vi "publishCurrentState.vi"(8 "error in (no error)":errorcluster, 11 "ElectrometerController in":refnum<class "ElectrometerController.lvclass">) -> (0 "error out":errorcluster, 3 "ElectrometerController out":refnum<class "ElectrometerController.lvclass">)   [LabVIEW 2016, in "ElectrometerController.lvclass"]
uses:
  ElectrometerController.lvclass
  ts_sallv_calibrationelectrometer/DataTypes/logevent_DetailedState.ctl
  ElectrometerController.lvclass/ElectrometerController.ctl
  ts_electrometeruserevents/PubSubDataEvent/PubSubDataEvent.lvclass/PubSubDataEvent.ctl
  Electrometer/State/ElectrometerState.lvclass
  ts_electrometeruserevents/PubSubDataEvent/PubSubDataEvent.lvclass
  ts_sallv_calibrationelectrometer/SALLV_calibrationElectrometer.lvlib
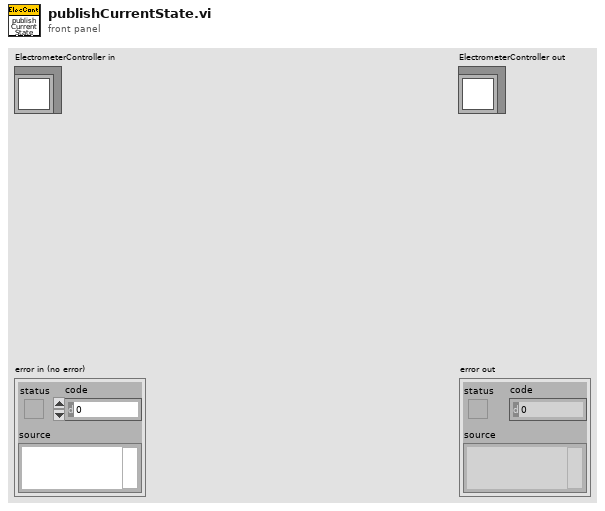
[diagram p1: front panel]
types:
  T1 = typedef "SALLV_calibrationElectrometer.lvlib/logevent_DetailedState.ctl" = cluster{"detailedState":u16, "electId":i16, "priority":i32}
  T2 = typedef "ElectrometerTypedefs.lvlib/PubDataEvents.ctl" = cluster{"ErrorCode":refnum<user-event>, "Heartbeat":refnum<user-event>, "LoopTime_ms":refnum<user-event>, "LoopTimeOutOfRange":refnum<user-event>, "RejectedCommand":refnum<user-event>, "SummaryState":refnum<user-event>, "Timestamp":refnum<user-event>, "AppliedSettingsMatchStart":refnum<user-event>, "InternalState":refnum<user-event>, "MeasureRange":refnum<user-event>, "DigitalFilterChange":refnum<user-event>, "IntensityReq":refnum<user-event>, "MeasureType":refnum<user-event>, "Intensity":refnum<user-event>, "IntegrationTime":refnum<user-event>, "SettingsAppliedSerialConfiguration":refnum<user-event>, "SettingsAppliedReadingSettings":refnum<user-event>, "SettingVersions":refnum<user-event>, "LargeFileObjectAvailable":refnum<user-event>, "DetailedState":refnum<user-event>}
  T3 = typedef "ElectrometerTypedefs.lvlib/StateValue.ctl" = enum16{"", "DisabledState", "EnabledState", "FaultState", "OffState", "StandbyState", "ReadyState", "ConfiguringState", "ManualReadingState", "UntilIntensityReadingState", "SetDurationReadingState", "BufferReadingState"}
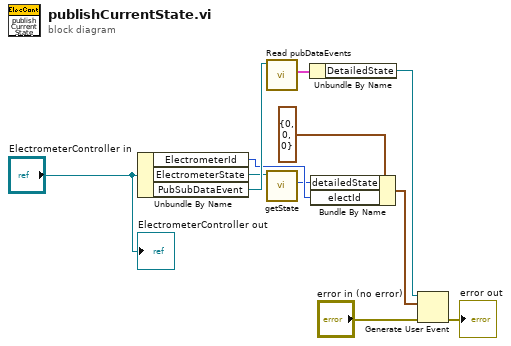
[diagram p0: block diagram]
diagram:
  n1 = Unbundle By Name("ElectrometerController in") -> ("ElectrometerId"=w3:enum16{"", "ID1", "ID2"}, "ElectrometerState"=w2:refnum<class "ElectrometerState.lvclass">, "PubSubDataEvent"=w10:refnum<class "PubSubDataEvent.lvclass">)
  n2 = call "Read pubDataEvents.vi"("PubSubDataEvent in"=w10) -> ("pubDataEvents"=w9:T2)  [unwired: 9 in, 1 out]
  n3 = call-dynamic "getState.vi"("State in"=w2) -> ("StateValue"=w1:T3)  [unwired: 8 in, 2 out]
  n4 = Unbundle By Name(w9) -> ("DetailedState"=w8:refnum<user-event>)
  n5 = Bundle By Name(cluster=T1 {"detailedState"=0, "electId"=0, "priority"=0} ("event data"), "detailedState"=w1, "electId"=w3) -> (w4:T1)
  n6 = Generate User Event(user event=w8, event data cluster=w4, error in="error in (no error)") -> (error out=→"error out":errorcluster)  [unwired: 1 in, 1 out]
  "ElectrometerController out" <- "ElectrometerController in"
